vi "Read.vi"(8 "error in (no error)":errorcluster, 10 "Timeout":u32, 11 "BaseDriver in":refnum<class "BaseDriver.lvclass">) -> (0 "error out":errorcluster, 3 "BaseDriver out":refnum<class "BaseDriver.lvclass">)   [LabVIEW 2013, in "BaseDriver.lvclass"]
doc: "Reads from the remote destination, handles and emits any response to the calling application"
uses:
  BaseDriver.lvclass
  BaseDriver.lvclass/BaseDriver.ctl
  Reader/BaseReader/BaseReader.lvclass
  driver_state.ctl
  Reader/BaseReader/BaseReader.lvclass/BaseReader.ctl
  Responder/BaseResponder/BaseResponder.lvclass
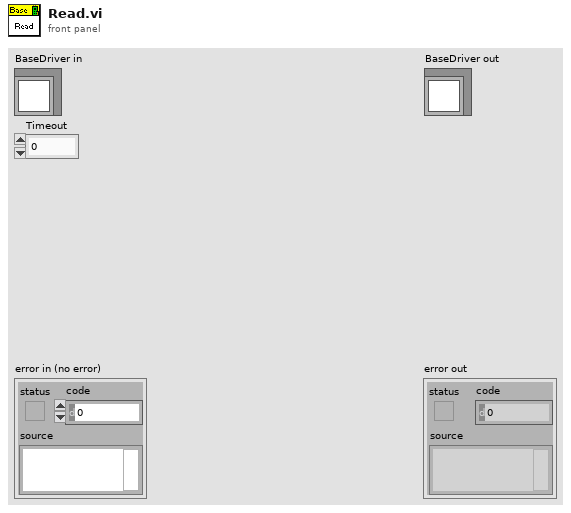
[diagram p1: front panel]
types:
  T1 = typedef "driver_state.ctl" = enum16{"Idle", "Wait for ack"}
  T2 = typedef "response.ctl" = cluster{"driver status":T3, "Sender":string, "Type":i32, "Variant":variant}
  T3 = typedef "driver_status.ctl" = enum16{"Normal", "Startup", "Connection lost", "Reconnected", "Timeout", "Idle", "Busy"}
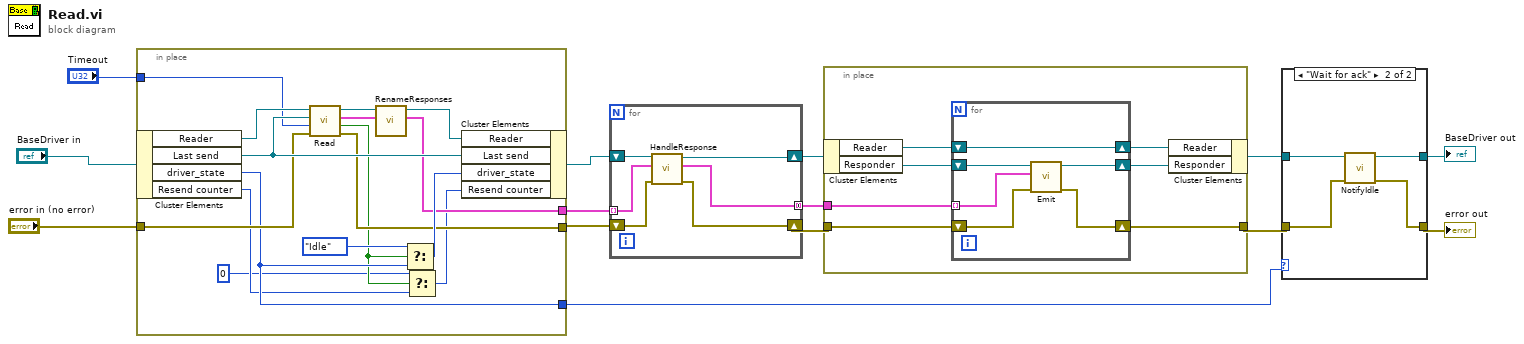
[diagram p0: block diagram]
diagram:
  n1 = in-place "In Place Element Structure" {
    in-place-border: [w19] -> w13
    in-place-border: "Timeout" -> [w26]
    in-place-border: "error in (no error)" -> [w25]
    in-place-border: [w24] -> w9
    in-place-border: [w23] -> w3
    n2 = in-place-cluster #1("BaseDriver in") -> ("Reader"=w29:refnum<class "BaseReader.lvclass">, "Last send"=w27:refnum<class "BaseMessage.lvclass">, "driver_state"=w23:T1, "Resend counter"=w18:i32)
    n3 = call-dynamic "Read.vi"("error in (no error)"=w25, "Timeout"=w26, "Last message"=w27, "BaseReader in"=w29) -> ("error out"=w24:errorcluster, "isAck?"=w17:bool, "Responses"=w20:T2[], "BaseReader out"=w22:refnum<class "BaseReader.lvclass">)  [unwired: 4 in]
    n4 = call "RenameResponses.vi"("Responses"=w20, "BaseReader in"=w22) -> ("Responses out"=w19:T2[], "BaseReader out"=w21:refnum<class "BaseReader.lvclass">)  [unwired: 7 in, 1 out]
    n5 = Select(t=driver_state."Idle" ("driver_state"), s=w17, f=w23) -> (s? t:f=w28:T1)
    n6 = Select(t=0, s=w17, f=w18) -> (s? t:f=w16:i32)
    n7 = in-place-cluster #1("Reader"=w21, "Last send"=w27, "driver_state"=w28, "Resend counter"=w16) -> (w14:refnum<class "BaseDriver.lvclass">)
  }
  n8 = for {
    shift-right: [w35] -> w12
    shift-left: w14 -> [w36]
    tunnel: w13 -> [w34] mode=indexing
    shift-right: [w32] -> w8
    shift-left: w9 -> [w33]
    tunnel: [w31] -> w1 mode=concatenating
    n9 = call-dynamic "HandleResponse.vi"("error in (no error)"=w33, "response"=w34, "BaseDriver in"=w36) -> ("error out"=w32:errorcluster, "Response out"=w31:T2[], "BaseDriver out"=w35:refnum<class "BaseDriver.lvclass">)  [unwired: 6 in]
  }
  n10 = in-place "In Place Element Structure" {
    in-place-border: w8 -> [w41]
    in-place-border: [w40] -> w5
    in-place-border: w1 -> [w37]
    n11 = in-place-cluster #2(w12) -> ("Reader"=w39:refnum<class "BaseReader.lvclass">, "Responder"=w43:refnum<class "BaseResponder.lvclass">)
    n12 = for {
      shift-right: [w48] -> w42
      shift-left: w43 -> [w49]
      tunnel: w37 -> [w45] mode=indexing
      shift-right: [w46] -> w40
      shift-left: w41 -> [w47]
      shift-right: [w44] -> w38
      shift-left: w39 -> [w44]
      n13 = call-dynamic "Emit.vi"("error in (no error)"=w47, "response"=w45, "BaseResponder in"=w49) -> ("error out"=w46:errorcluster, "BaseResponder out"=w48:refnum<class "BaseResponder.lvclass">)  [unwired: 7 in]
    }
    n14 = in-place-cluster #2("Reader"=w38, "Responder"=w42) -> (w7:refnum<class "BaseDriver.lvclass">)
  }
  n15 = case shown="\"Wait for ack\"" w3 {
    tunnel: w7 -> [w51 w55]
    tunnel: [w51 w54] -> w6
    tunnel: w5 -> [w50 w53]
    tunnel: [w50 w52] -> w4
    frame "Idle", Default {
    }
    frame "Wait for ack" {
      n16 = call "NotifyIdle.vi"("error in (no error)"=w53, "BaseDriver in"=w55) -> ("error out"=w52:errorcluster, "BaseDriver out"=w54:refnum<class "BaseDriver.lvclass">)  [unwired: 8 in]
    }
  }
  "error out" <- w4
  "BaseDriver out" <- w6
